vi "enable_burst.vi"(0 "VISA resource name":refnum<visa-resource-name>="TRIG", 3 "error in (no error)":errorcluster, 4 "Burst enable?":bool) -> (5 "VISA resource name out":refnum<visa-resource-name>, 7 "error out":errorcluster)   [LabVIEW 2011]
doc: "Sets he burst period and the burst count. \n\nSets he burst count. When burst mode is enabled, the DG645 \noutputs burst count delay cycles per trigger.\n\nThe burst period sets the time between delay cycles during a burst. \nThe burst period may range from 100 ns to 2000 – 10 ns in 10 ns steps."
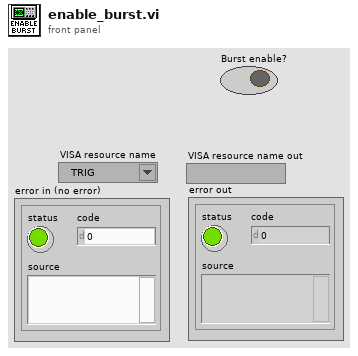
[diagram p1: front panel]
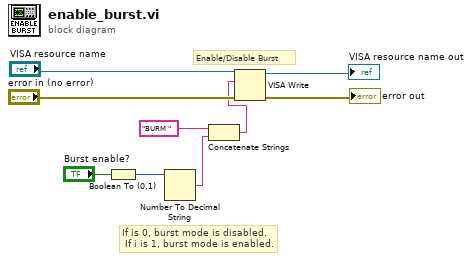
[diagram p0: block diagram]
diagram:
  # "Enable/Disable Burst"
  # "If is 0, burst mode is disabled.\n If i is 1, burst mode is enabled."
  n1 = Boolean To (0,1)(Boolean="Burst enable?") -> (0, 1=w4:i16)
  n2 = Number To Decimal String(number=w4) -> (decimal integer string=w3:string)  [unwired: 1 in]
  n3 = Concatenate Strings("BURM " ("Query 2"), w3) -> (w5:string)
  n4 = VISA Write(VISA resource name="VISA resource name", write buffer=w5, error in (no error)="error in (no error)") -> (VISA resource name out=→"VISA resource name out":refnum<visa-resource-name>, error out=→"error out":errorcluster)  [unwired: 1 out]
